vi "read forward power out dBm.vi"() -> ()   [LabVIEW 2009]
panel:
  out "result string":string
  out "VISA resource name out":refnum<visa-resource-name>
  in  "VISA resource name":refnum<visa-resource-name>="GPIB0::12::INSTR"
  in  "error in (no error)":errorcluster
  out "read buffer":string
  in  "read? (f)":bool=TRUE
  in  "bytes to read (1000)":u32=1000
  out "bytes read":u32
  out "error out":errorcluster
  in  "write buffer":string="RDPOD"
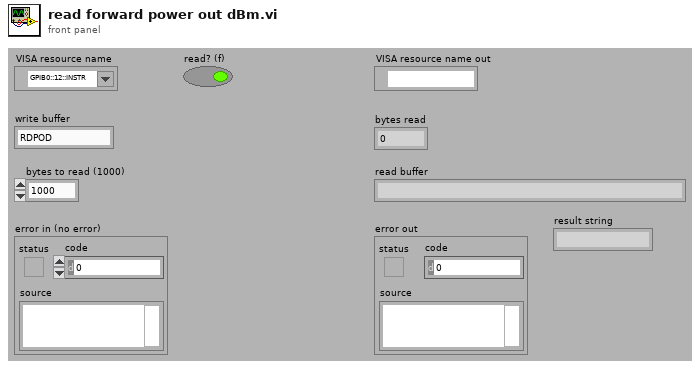
[diagram p1: front panel]
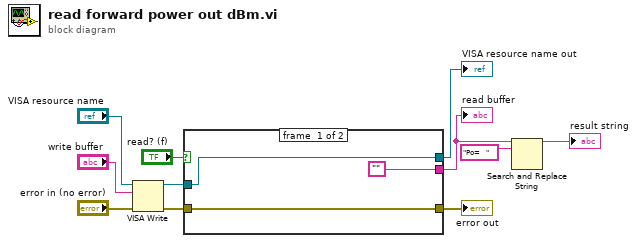
[diagram p0: block diagram]
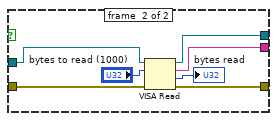
[diagram p2: hidden frame]
diagram:
  n1 = VISA Write(VISA resource name="VISA resource name", write buffer="write buffer", error in (no error)="error in (no error)") -> (VISA resource name out=w5:refnum<visa-resource-name>, error out=w4:errorcluster)  [unwired: 1 out]
  n2 = case shown="True" "read? (f)" {
    tunnel: w4 -> [w13 w15]
    tunnel: [w13 w21] -> w8
    tunnel: [w14 w19] -> w7
    tunnel: w5 -> [w14 w16]
    tunnel: ["" w18] -> w1
    frame #0 {
    }
    frame #1 {
      n3 = VISA Read(VISA resource name=w16, byte count="bytes to read (1000)", error in (no error)=w15) -> (VISA resource name out=w19:refnum<visa-resource-name>, read buffer=w18:string, return count=→"bytes read":u32, error out=w21:errorcluster)
    }
  }
  "error out" <- w8
  "read buffer" <- w1
  "VISA resource name out" <- w7
  n4 = Search and Replace String(input string=w1, search string="Po=   ") -> (result string=→"result string":string)  [unwired: 6 in, 3 out]
